vi "BUILD_install for dependencies core.vi"(6 "buildlog":path, 8 "error in":errorcluster, 9 "args":string[](array[string]), 11 "vipb path":path) -> (0 "error out":errorcluster)   [LabVIEW 2010]
uses:
  <vilib>/JKI/VIPM API/VIPM API_vipm_api.lvlib
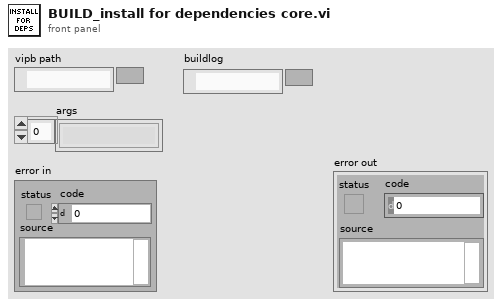
[diagram p1: front panel]
types:
  T1 = typedef "VIPM API_vipm_api.lvlib/Library Contents Cluster_vipm_api.ctl" = cluster{"Package Name":string, "Version":string, "Display Name":string, "Repository Name":string, "Company Name":string, "License Type":string, "Installed":bool, "Deprecated":bool, "Dependency or Conflict Problem":bool, "Downloaded":bool}
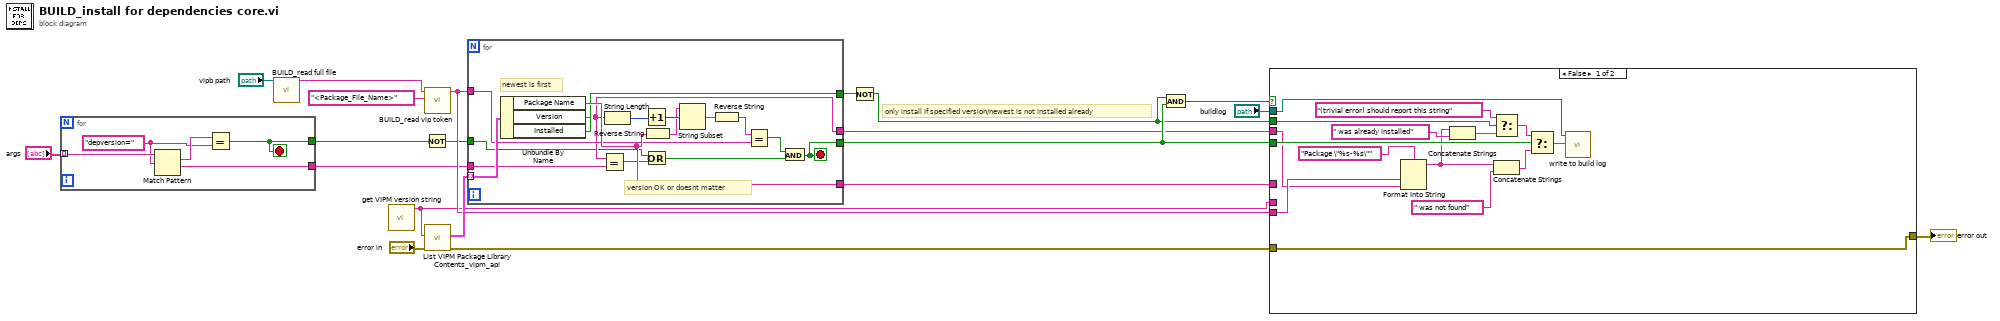
[diagram p0: block diagram]
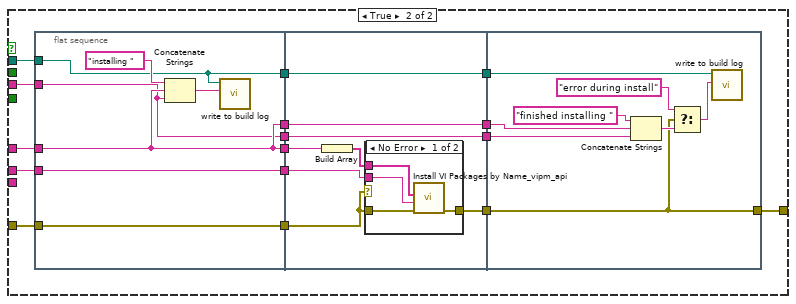
[diagram p2: hidden frame]
diagram:
  # "only install if specified version/newest is not installed already"
  n1 = for {
    tunnel: "args" -> [w25] mode=indexing
    tunnel: [w22] -> w3
    tunnel: [w21] -> w2
    stop <- w21 stop-if-true
    w23 = "depversion=" ("regular expression")
    n2 = Match Pattern(string=w25, regular expression=w23) -> (match substring=w24:string, after substring=w22:string)  [unwired: 1 in, 2 out]
    n3 = Equal?(x=w24, y=w23) -> (x = y?=w21:bool)
  }
  n4 = call "BUILD_read full file.vi"("vip file"="vipb path") -> ("data"=w19:string)  [unwired: 9 in, 1 out]
  n5 = call "get VIPM version string.vi"() -> ("version string"=w5:string)  [unwired: 11 in]
  n6 = Not(x=w2) -> (.not. x?=w1:bool)
  n7 = call "BUILD_read vip token.vi"("regular expression"="<Package_File_Name>", "data"=w19) -> ("trimmed string"=w7:string)  [unwired: 9 in]
  n8 = call <vilib>:"List VIPM Package Library Contents_vipm_api.vi"("error in (no error)"="error in", "LabVIEW Version"=w5) -> ("error out"=w17:errorcluster, "Library Contents []"=w16:T1[])  [unwired: 8 in]
  n9 = for {
    tunnel: w16 -> [w41] mode=indexing
    tunnel: [w36] -> w18
    tunnel: [w27] -> w9
    tunnel: w7 -> [w33]
    tunnel: [w32] -> w12
    tunnel: [w30] -> w4
    tunnel: w3 -> [w31]
    tunnel: w1 -> [w28]
    stop <- w27 stop-if-true
    # "version OK or doesnt matter"
    # "newest is first"
    n10 = Unbundle By Name(w41) -> ("Package Name"=w36:string, "Version"=w30:string, "Installed"=w32:bool)
    n11 = Equal?(x=w30, y=w31) -> (x = y?=w29:bool)
    n12 = String Length(string=w30) -> (length=w40:i32)
    n13 = Increment(x=w40) -> (x+1=w39:i32)
    n14 = Or(x=w28, y=w29) -> (x .or. y?=w26:bool)
    n15 = Reverse String(1:w36) -> (0:w38:string)
    n16 = String Subset(string=w38, offset (0)=w39) -> (substring=w37:string)  [unwired: 1 in]
    n17 = Reverse String(1:w37) -> (0:w35:string)
    n18 = Equal?(x=w35, y=w33) -> (x = y?=w34:bool)
    n19 = And(x=w34, y=w26) -> (x .and. y?=w27:bool)
  }
  n20 = Not(x=w12) -> (.not. x?=w8:bool)
  n21 = And(x=w8, y=w9) -> (x .and. y?=w13:bool)
  n22 = case shown="False" w13 {
    tunnel: [w56 w70] -> w14
    tunnel: w5 -> [_ w71]
    tunnel: w17 -> [w56 w69]
    tunnel: w18 -> [_ w72]
    tunnel: "buildlog" -> [w55 w64]
    tunnel: w9 -> [w54 _]
    tunnel: w8 -> [w49 _]
    tunnel: w7 -> [w53 _]
    tunnel: w4 -> [w42 w59]
    frame False {
      n23 = Format Into String(format string="Package \"%s-%s\"", w53, w42) -> (resulting string=w46:string)  [unwired: 2 in, 1 out]
      n24 = Concatenate Strings(w46, " was already installed" ("string")) -> (w45:string)
      n25 = Select(t="(trivial error) should report this string", s=w49, f=w45) -> (s? t:f=w44:string)
      n26 = Concatenate Strings(w46, " was not found" ("string")) -> (w51:string)
      n27 = Select(t=w44, s=w54, f=w51) -> (s? t:f=w48:string)
      n28 = call "write to build log.vi"("text"=w48, "log"=w55) -> ()  [unwired: 10 in]
    }
    frame True {
      n29 = flat-sequence {
        tunnel: w69 -> [w78]
        tunnel: w71 -> [w79]
        tunnel: w72 -> [w74]
        tunnel: [w74] -> w67
        tunnel: [w79] -> w66
        tunnel: [w78] -> w65
        tunnel: w64 -> [w75]
        tunnel: [w75] -> w62
        tunnel: [w74] -> w61
        tunnel: w59 -> [w73]
        tunnel: [w73] -> w58
        tunnel: [w84] -> w68
        tunnel: w67 -> [w87]
        tunnel: w66 -> [w85]
        tunnel: w65 -> [w83]
        tunnel: [w82] -> w63
        tunnel: w62 -> [w82]
        tunnel: w61 -> [w81]
        tunnel: [w81] -> w60
        tunnel: w58 -> [w80]
        tunnel: [w80] -> w57
        tunnel: [w95] -> w70
        tunnel: w68 -> [w95]
        tunnel: w63 -> [w99]
        tunnel: w60 -> [w98]
        tunnel: w57 -> [w93]
        frame #0 {
          n30 = Concatenate Strings("installing " ("string"), w74, w73) -> (w76:string)
          n31 = call "write to build log.vi"("text"=w76, "log"=w75) -> ()  [unwired: 10 in]
        }
        frame #1 {
          n32 = Build Array(w87) -> (w86:string[])
          n33 = case shown="No Error" w83 {
            tunnel: w86 -> [w91 _]
            tunnel: w85 -> [w90 _]
            tunnel: w83 -> [w89 w92]
            tunnel: [w88 w92] -> w84
            frame No Error {
              n34 = call <vilib>:"Install VI Packages by Name_vipm_api.vi"("error in (no error)"=w89, "LabVIEW Version"=w90, "Package Names to Install []"=w91) -> ("error out"=w88:errorcluster)  [unwired: 8 in]
            }
            frame Error {
            }
          }
        }
        frame #2 {
          n35 = Concatenate Strings("finished installing " ("string"), w98, w93) -> (w97:string)
          n36 = Select(t="error during install", s=w95, f=w97) -> (s? t:f=w96:string)
          n37 = call "write to build log.vi"("text"=w96, "log"=w99) -> ()  [unwired: 10 in]
        }
      }
    }
  }
  "error out" <- w14
